vi "Set Simulated.vi"(8 "error in (no error)":errorcluster, 10 "Simulated":bool, 11 "PS in":refnum<class "PS.lvclass">) -> (0 "error out":errorcluster, 3 "PS out":refnum<class "PS.lvclass">)   [LabVIEW 2021, in "PS.lvlib" / "PS.lvclass"]
uses:
  PS.lvclass
  PS.lvclass/PS.ctl
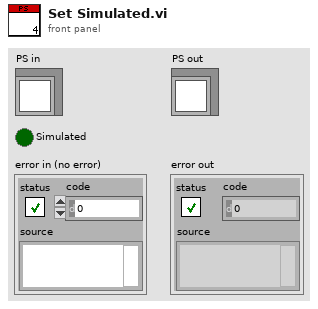
[diagram p1: front panel]
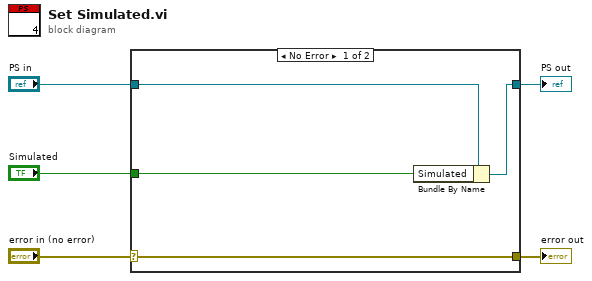
[diagram p0: block diagram]
diagram:
  n1 = case shown="No Error" "error in (no error)" {
    selector: "error in (no error)" -> [w9 w10]
    tunnel: [w9 w10] -> w4
    tunnel: [w7 w11] -> w2
    tunnel: "PS in" -> [w8 w11]
    tunnel: "Simulated" -> [w6 _]
    frame No Error {
      n2 = Bundle By Name(cluster=w8, "Simulated"=w6) -> (w7:refnum<class "PS.lvclass">)
    }
    frame Error {
    }
  }
  "error out" <- w4
  "PS out" <- w2
